vi "Build Json.vi"(8 "Error In":errorcluster, 11 "Asset":refnum<class "Asset.lvclass">) -> (0 "Error Out":errorcluster, 2 "JSON File Content":string, 3 "JSON File Name":string)   [LabVIEW 2019, in "Asset.lvclass"]
uses:
  Asset.lvclass
  AssetJson.ctl
  AssetLocationJson.ctl
  AssetExternalCalibrationJson.ctl
  ExternalCalibrationOperatorJson.ctl
  AssetsJson.ctl
  Asset Location/Asset Location.lvclass
  Asset External Calibration/Asset External Calibration.lvclass
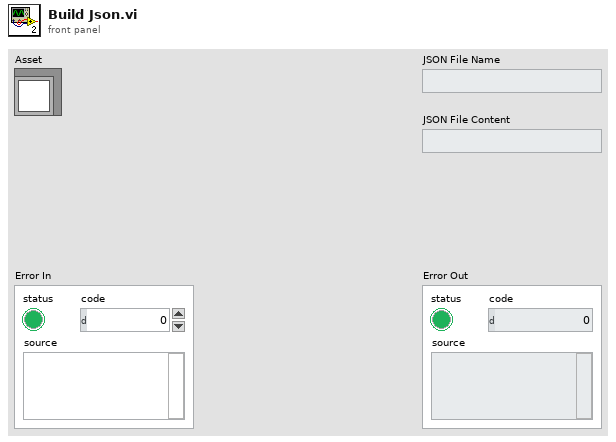
[diagram p1: front panel]
types:
  T1 = typedef "Asset.lvclass/AssetsJson.ctl" = cluster{"assets":T2[]}
  T2 = typedef "Asset.lvclass/AssetJson.ctl" = cluster{"serialNumber":string, "modelName":string, "modelNumber":u32, "vendorName":string, "vendorNumber":u32, "busType":string, "assetClass":string, "assetName":string, "firmwareVersion":string, "hardwareVersion":string, "location":T3, "supportsExternalCalibration":bool, "externalCalibration":T4}
  T3 = typedef "Asset.lvclass/AssetLocationJson.ctl" = cluster{"slotNumber":u32, "parent":string}
  T4 = typedef "Asset.lvclass/AssetExternalCalibrationJson.ctl" = cluster{"date":string, "comments":string, "recommendedInterval":u32, "operator":T5}
  T5 = typedef "Asset.lvclass/ExternalCalibrationOperatorJson.ctl" = cluster{"displayName":string, "userId":string}
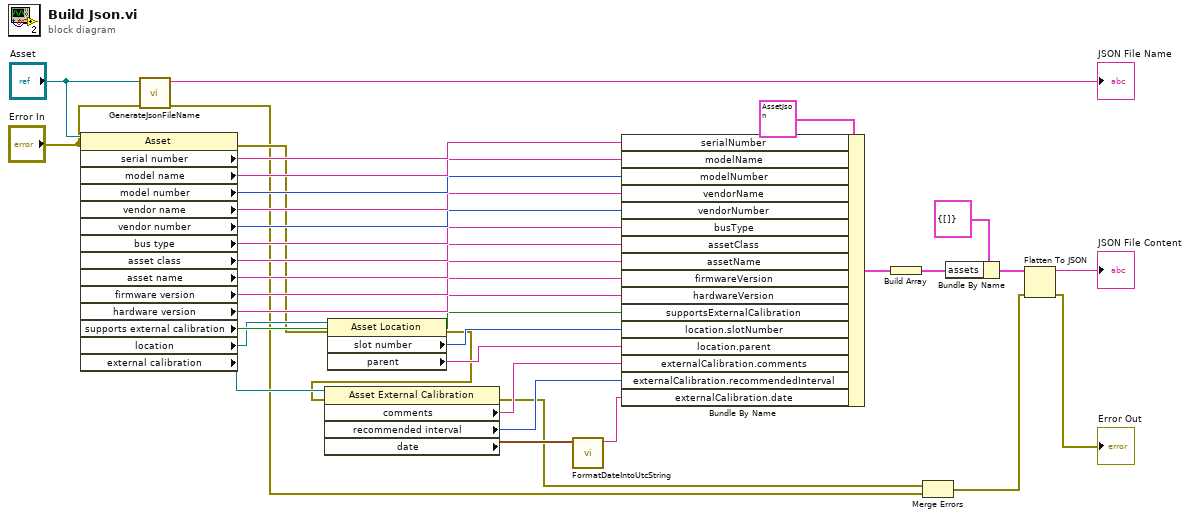
[diagram p0: block diagram]
diagram:
  n1 = property class="Asset"(reference="Asset", error in="Error In") -> (error out=w11:errorcluster, "serial number"=w34:string, "model name"=w33:string, "model number"=w32:u32, "vendor name"=w31:string, "vendor number"=w30:u32, "bus type"=w29:string, "asset class"=w28:string, "asset name"=w27:string, "firmware version"=w26:string, "hardware version"=w25:string, "supports external calibration"=w19:bool, "location"=w18:refnum<class "Asset Location.lvclass">, "external calibration"=w24:refnum<class "Asset External Calibration.lvclass">)  [unwired: 1 out]
  n2 = call "GenerateJsonFileName.vi"("Error In"="Error In", "Asset"="Asset") -> ("Error Out"=w9:errorcluster, "File Name"=→"JSON File Name":string)  [unwired: 8 in]
  n3 = property class="Asset Location"(reference=w18, error in=w11) -> (error out=w5:errorcluster, "slot number"=w17:u32, "parent"=w16:string)  [unwired: 1 out]
  n4 = property class="Asset External Calibration"(reference=w24, error in=w5) -> (error out=w10:errorcluster, "comments"=w14:string, "recommended interval"=w13:u32, "date"=w15:timestamp)  [unwired: 1 out]
  n5 = call "FormatDateIntoUtcString.vi"("Date (UTC)"=w15) -> ("Formatted Date (UTC)"=w12:string)  [unwired: 10 in]
  n6 = Bundle By Name(cluster=T2 {"serialNumber"="", "modelName"="", "modelNumber"=0, "vendorName"="", "vendorNumber"=0, "busType"="", "assetClass"="", "assetName"="", "firmwareVersion"="", "hardwareVersion"="", "location"={"slotNumber"=0, "parent"=""}, "supportsExternalCalibration"=FALSE, "externalCalibration"={"date"="", "comments"="", "recommendedInterval"=0, "operator"={"displayName"="", "userId"=""}}} ("Asset"), "serialNumber"=w34, "modelName"=w33, "modelNumber"=w32, "vendorName"=w31, "vendorNumber"=w30, "busType"=w29, "assetClass"=w28, "assetName"=w27, "firmwareVersion"=w26, "hardwareVersion"=w25, "supportsExternalCalibration"=w19, "location.slotNumber"=w17, "location.parent"=w16, "externalCalibration.comments"=w14, "externalCalibration.recommendedInterval"=w13, "externalCalibration.date"=w12) -> (w2:T2)
  n7 = Build Array(w2) -> (w1:T2[])
  n8 = Merge Errors(w10, w9) -> (w4:errorcluster)
  n9 = Bundle By Name(cluster=T1 {"assets"=[]} ("json"), "assets"=w1) -> (w6:T1)
  n10 = Flatten To JSON(anything=w6, error in (no error)=w4) -> (JSON string=→"JSON File Content":string, 11:→"Error Out":errorcluster)  [unwired: 1 in]
